vi "Modbus Data Massage.vi"(1 "register values":u16[][](array[numeric]), 2 "Modbus Req":T1) -> (0 "Output Data":dbl[](array[numeric]))   [LabVIEW 2020]
uses:
  Control/Device Name.ctl
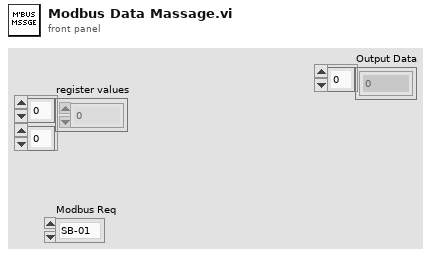
[diagram p1: front panel]
types:
  T1 = typedef "Device Name.ctl" = enum16{"SB-01", "SB-02", "BANK-01", "BANK-02", "SI-M", "SI-01", "PM-01"}
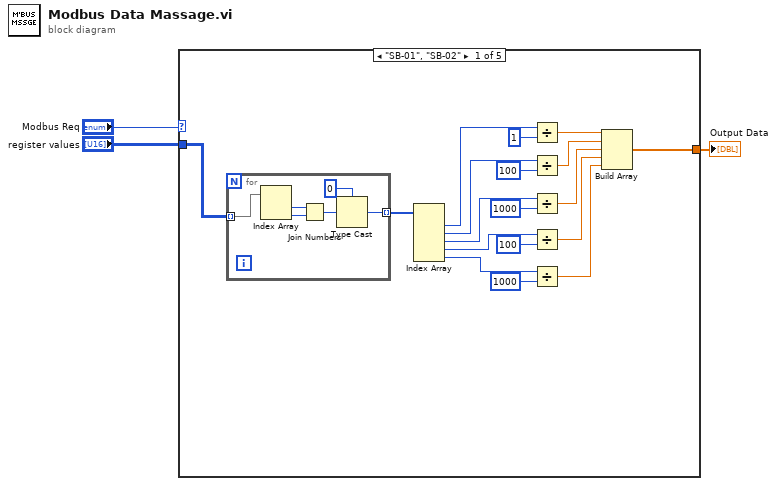
[diagram p0: block diagram]
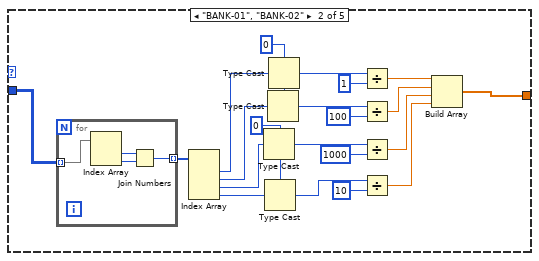
[diagram p2: hidden frame]
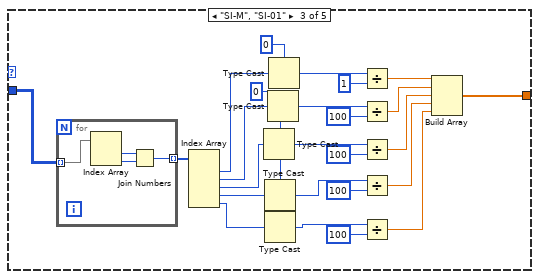
[diagram p3: hidden frame]
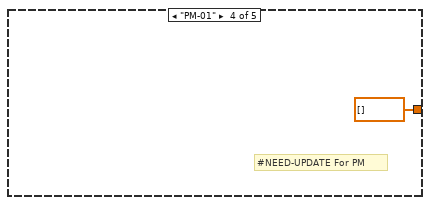
[diagram p4: hidden frame]
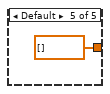
[diagram p5: hidden frame]
diagram:
  n1 = case shown="\"SB-01\", \"SB-02\"" "Modbus Req" {
    tunnel: "register values" -> [w21 w48 w77 _ _]
    tunnel: [w4 w34 w63 dbl[] [] dbl[] []] -> w1
    frame "SB-01", "SB-02" {
      n2 = for {
        tunnel: w21 -> [w27] mode=indexing
        tunnel: [w23] -> w20 mode=indexing
        n3 = Index Array(array=w27) -> (element #1=w26:u16, element #2=w25:u16)  [unwired: 2 in]
        n4 = Join Numbers(hi=w26, lo=w25) -> ((hi.lo)=w24:u32)
        n5 = Type Cast(type=0, x=w24) -> (*(type *) &x=w23:i32)
      }
      n6 = Index Array(array=w20) -> (element #1=w19:i32, element #2=w17:i32, element #3=w15:i32, element #4=w13:i32, element #5=w11:i32)  [unwired: 5 in]
      n7 = Divide(x=w19, y=1) -> (x/y=w9:dbl)
      n8 = Divide(x=w17, y=100) -> (x/y=w8:dbl)
      n9 = Divide(x=w15, y=1000) -> (x/y=w7:dbl)
      n10 = Divide(x=w13, y=100) -> (x/y=w6:dbl)
      n11 = Divide(x=w11, y=1000) -> (x/y=w5:dbl)
      n12 = Build Array(w9, w8, w7, w6, w5) -> (w4:dbl[])
    }
    frame "BANK-01", "BANK-02" {
      w28 = 0
      w31 = u32 0
      n13 = for {
        tunnel: w48 -> [w52] mode=indexing
        tunnel: [w49] -> w47 mode=indexing
        n14 = Index Array(array=w52) -> (element #1=w51:u16, element #2=w50:u16)  [unwired: 2 in]
        n15 = Join Numbers(hi=w51, lo=w50) -> ((hi.lo)=w49:u32)
      }
      n16 = Index Array(array=w47) -> (element #1=w46:u32, element #2=w44:u32, element #3=w42:u32, element #4=w40:u32)  [unwired: 4 in]
      n17 = Type Cast(type=w28, x=w42) -> (*(type *) &x=w30:i32)
      n18 = Type Cast(type=w28, x=w40) -> (*(type *) &x=w29:i32)
      n19 = Type Cast(type=w31, x=w44) -> (*(type *) &x=w32:u32)
      n20 = Type Cast(type=w31, x=w46) -> (*(type *) &x=w33:u32)
      n21 = Divide(x=w33, y=1) -> (x/y=w38:dbl)
      n22 = Divide(x=w32, y=100) -> (x/y=w37:dbl)
      n23 = Divide(x=w30, y=1000) -> (x/y=w36:dbl)
      n24 = Divide(x=w29, y=10) -> (x/y=w35:dbl)
      n25 = Build Array(w38, w37, w36, w35) -> (w34:dbl[])
    }
    frame "SI-M", "SI-01" {
      w57 = 0
      n26 = for {
        tunnel: w77 -> [w81] mode=indexing
        tunnel: [w78] -> w76 mode=indexing
        n27 = Index Array(array=w81) -> (element #1=w80:u16, element #2=w79:u16)  [unwired: 2 in]
        n28 = Join Numbers(hi=w80, lo=w79) -> ((hi.lo)=w78:u32)
      }
      n29 = Index Array(array=w76) -> (element #1=w75:u32, element #2=w73:u32, element #3=w71:u32, element #4=w69:u32, element #5=w56:u32)  [unwired: 5 in]
      n30 = Type Cast(type=w57, x=w71) -> (*(type *) &x=w59:i32)
      n31 = Type Cast(type=w57, x=w69) -> (*(type *) &x=w58:i32)
      n32 = Type Cast(type=w57, x=w56) -> (*(type *) &x=w54:i32)
      n33 = Type Cast(type=w57, x=w73) -> (*(type *) &x=w61:i32)
      n34 = Type Cast(type=u32 0, x=w75) -> (*(type *) &x=w62:u32)
      n35 = Divide(x=w62, y=1) -> (x/y=w67:dbl)
      n36 = Divide(x=w61, y=100) -> (x/y=w66:dbl)
      n37 = Divide(x=w59, y=100) -> (x/y=w65:dbl)
      n38 = Divide(x=w58, y=100) -> (x/y=w64:dbl)
      n39 = Divide(x=w54, y=100) -> (x/y=w53:dbl)
      n40 = Build Array(w67, w66, w65, w64, w53) -> (w63:dbl[])
    }
    frame "PM-01" {
      # "#NEED-UPDATE For PM"
    }
    frame Default {
    }
  }
  "Output Data" <- w1
